vi "Deadband.vi"(8 "Totbereich -":sgl, 9 "Totbereich +":sgl, 11 "Ausgang":sgl) -> (3 "Ausgang":sgl)   [LabVIEW 2020, in "Regler.lvlib" / "Druckregler.lvlib"]
uses:
  Druckregler.lvlib
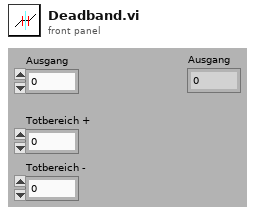
[diagram p1: front panel]
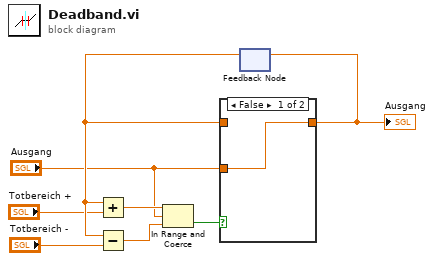
[diagram p0: block diagram]
diagram:
  n1 = feedback #1() -> (w7:sgl)  [unwired: 1 in]
  n2 = Add(x=w7, y="Totbereich +") -> (x+y=w2:sgl)
  n3 = Subtract(x=w7, y="Totbereich -") -> (x-y=w4:sgl)
  n4 = In Range and Coerce(upper limit=w2, x="Ausgang", lower limit=w4) -> (In Range?=w6:bool)  [unwired: 1 out]
  n5 = case shown="False" w6 {
    tunnel: "Ausgang" -> [w9 _]
    tunnel: w7 -> [_ w10]
    tunnel: [w9 w10] -> w8
    frame False {
    }
    frame True {
    }
  }
  "Ausgang" <- w8
  n6 = feedback-in #1(w8) -> ()
